vi "OAT Add Orbit Plot Label.vi"(5 "plot type":u16(ring) items=["unfiltered", "filtered"], 6 "max value":dbl format="%.2f", 7 "orbit plot ref":refnum<vi>, 8 "error in (no error)":errorcluster, 9 "probe angle out":cluster{"X (red)":dbl, "Y (blue)":dbl}, 10 "orbit precession direction":u16(ring) items=["forward", "backward"], 11 "XY plot data in":cluster{dbl[], dbl[]}[](array[cluster]) {"?" format="%.2f"; "?" format="%.2f"}) -> (0 "error out":errorcluster, 3 "XY plot data out":cluster{dbl[], dbl[]}[](array[cluster]) {"?" format="%.2f"; "?" format="%.2f"})   [LabVIEW 2017]
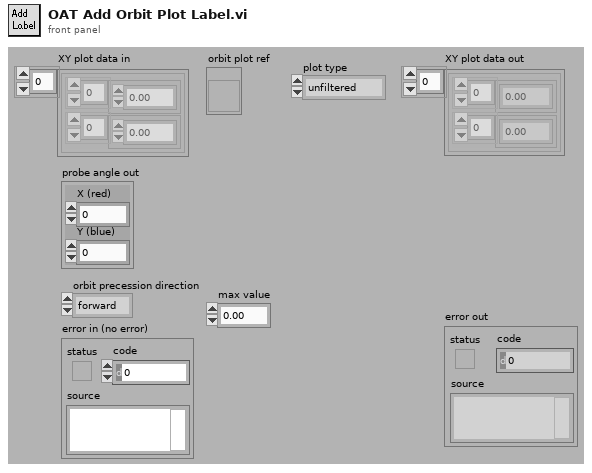
[diagram p1: front panel]
types:
  T1 = cluster{"Name":string, "Color":u32, "Hair Style":u8, "Point Style":u8, "Name Visible":bool, "Trackable":bool, "Lock Style":u32, "Plot Number":u32, "Marker Index":i32, "Location":cluster{"X":dbl, "Y":dbl}}
  T2 = cluster{"Name":string, "Color":u32, "Hair Style":u8, "Point Style":u8, "Name Visible":bool, "Trackable":bool, "Lock Style":u32, "Plot Number":u32, "Marker Index":i32, "Location":cluster{"X":dbl, "Y":dbl}}[]
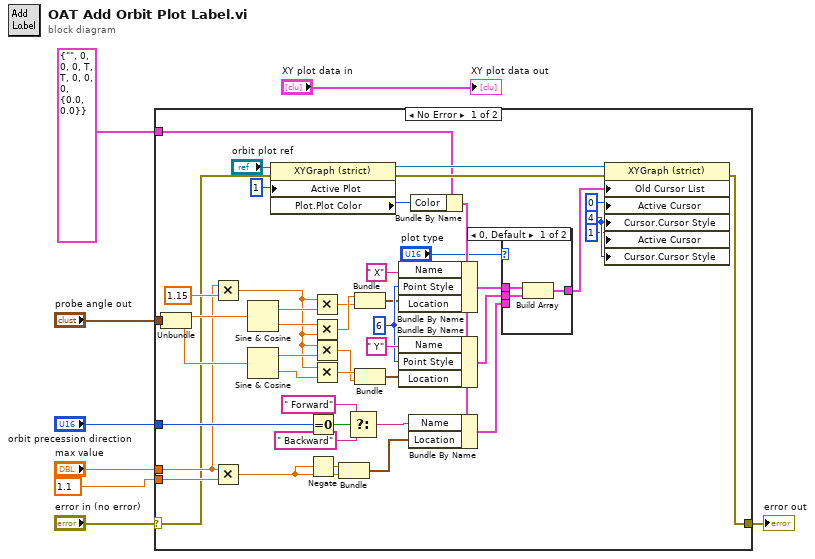
[diagram p0: block diagram]
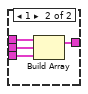
[diagram p2: hidden frame]
diagram:
  n1 = case shown="No Error" "error in (no error)" {
    selector: "error in (no error)" -> [w10 w61]
    tunnel: 1.1 ("y") -> [w53 _]
    tunnel: "orbit precession direction" -> [w52 _]
    tunnel: "probe angle out" -> [w38 _]
    tunnel: T1 {"Name"="", "Color"=0, "Hair Style"=0, "Point Style"=0, "Name Visible"=TRUE, "Trackable"=TRUE, "Lock Style"=0, "Plot Number"=0, "Marker Index"=0, "Location"={"X"=0.0, "Y"=0.0}} -> [w16 _]
    tunnel: "max value" -> [w13 _]
    tunnel: [w9 w61] -> w1
    frame No Error {
      w39 = u8 4 ("Cursor.Cursor Style")
      w40 = u8 6 ("Point Style")
      n2 = Unbundle(w38) -> ("X (red)"=w21:dbl, "Y (blue)"=w22:dbl)
      n3 = Multiply(x=w13, y=1.15) -> (x*y=w23:dbl)
      n4 = Multiply(x=w13, y=w53) -> (x*y=w25:dbl)
      n5 = Sine & Cosine(0:w21) -> (1:w31:dbl, 2:w32:dbl)
      n6 = Sine & Cosine(0:w22) -> (1:w37:dbl, 2:w36:dbl)
      n7 = property class="XYGraph (strict)"(reference="orbit plot ref", error in=w10, "Active Plot"=u32 1) -> (reference out=w19:refnum<vi>, error out=w18:errorcluster, "Plot.Plot Color"=w14:u32)
      n8 = Equal To 0?(x=w52) -> (x = 0?=w51:bool)
      n9 = Negate(x=w25) -> (-x=w48:dbl)
      n10 = Multiply(x=w23, y=w31) -> (x*y=w29:dbl)
      n11 = Multiply(x=w32, y=w23) -> (x*y=w30:dbl)
      n12 = Multiply(x=w23, y=w37) -> (x*y=w34:dbl)
      n13 = Multiply(x=w23, y=w36) -> (x*y=w35:dbl)
      n14 = Bundle(w48, w25) -> (w45:cluster{dbl, dbl})  [unwired: 1 in]
      n15 = Select(t=" Forward", s=w51, f=" Backward") -> (s? t:f=w46:string)
      n16 = Bundle(w30, w29) -> (w28:cluster{dbl, dbl})  [unwired: 1 in]
      n17 = Bundle(w35, w34) -> (w33:cluster{dbl, dbl})  [unwired: 1 in]
      n18 = Bundle By Name(cluster=w16, "Color"=w14) -> (w15:T1)
      n19 = Bundle By Name(cluster=w15, "Name"=" X", "Point Style"=w40, "Location"=w28) -> (w43:T1)
      n20 = Bundle By Name(cluster=w15, "Name"=" Y", "Point Style"=w40, "Location"=w33) -> (w41:T1)
      n21 = Bundle By Name(cluster=w15, "Name"=w46, "Location"=w45) -> (w12:T1)
      n22 = case shown="0, Default" "plot type" {
        tunnel: [w54 w60] -> w47
        tunnel: w43 -> [w56 w59]
        tunnel: w41 -> [w55 w58]
        tunnel: w12 -> [_ w57]
        frame 0, Default {
          n23 = Build Array(w56, w55) -> (w54:T2)
        }
        frame 1 {
          n24 = Build Array(w59, w58, w57) -> (w60:T2)
        }
      }
      n25 = property class="XYGraph (strict)"(reference=w19, error in=w18, "Old Cursor List"=w47, "Active Cursor"=u32 0, "Cursor.Cursor Style"=w39, "Active Cursor"=u32 1, "Cursor.Cursor Style"=w39) -> (error out=w9:errorcluster)  [unwired: 1 out]
    }
    frame Error {
    }
  }
  "error out" <- w1
  "XY plot data out" <- "XY plot data in"
